vi "Puma_Ground_Control_Station_V2.0.vi"(0 "?":refnum<visa-resource-name>="COM4", 1 "?":u32=9600, 9 "XON":u8=17 format="%.0x", 14 "XOFF":u8=19 format="%.0x", 15 "?":u32=10000, 21 "?":bool=TRUE, 24 "?":u8=10 format="%.0x", 25 "bsize":u32=4096) -> ()   [LabVIEW 2015]
doc: "The Advanced Serial Read and Write example performs a Serial Port Read, a Serial Port Write, or a combination of these actions while setting some advanced serial features like buffer size, termination characters, and XON/XOFF flow control. The user selects the actions (read or write) on the front panel. If both are selected, the VI will write the data first, read the data and then close the VISA session that is opened to the port. \n\nThe parameters set for the serial port must match the parameters of the connected instrument or device. In this example, the bytes to read parameter specifies the number of bytes that the serial port reads. If there were more bytes at the port than the number specified in bytes to read, those bytes would not be read. Also, if you specify to read more bytes than the number of bytes actually read, you might receive a timeout error message.\n\nINSTRUCTIONS:\n1) Select the serial resource and configuration parameters (baud rate, data bits, parity, stop bits, flow control).\n2) Termination character can be enabled and set. Also, set the required input buffer size prior to running the example.\n3) Select the operations to be performed. \n4) Connect the serial port to your device. If no device is available, perform a loopback test by doing one of the following. Short pins 2 and 3 on a RS-232 cable or short pin 4 to pin 8 and pin 5 to pin 9 on a RS-485/422 cable. \n5) Run the VI to see the data read. (The \"read string\" will match the \"string to write\" if a loopback test was performed.)\n\nThis example exposes several advanced features that you may need for your application. Not all applications need all the features shown in this example. The input buffer size is likely an important setting that you want to control in your application. This example expands upon the flow control option for XON and XOFF, allowing the user to choose those control characters. The timeout parameter has been brought to the front panel so a user can specify the time period the VISA Read will wait for the number of bytes to read before timing out. Also, the user has several controls for the termination character, which is discussed later.\n\nNote that you can press the write and read buttons and change the bytes to read parameters on the fly, while the example is running. However, you must stop the example to change the other configuration parameters after the example has started running, and then run again.\n\nSet the I/O buffer size slightly higher the amount of data you expect to receive. This is very important for applications that don't use flow control, as you may lose characters if the receive buffer overflows.\n\nSetting the timeout period ensures that the operation returns with a timeout error if the operation cannot be performed in the specified time period. \n\nSome devices require a termination character in order to identify the end of command strings. Some devices send a termination character to signify the end of data to be read. \n\nThis example shows how you can end the Read operation once a termination character is detected in the buffer and/or append a termination character at the end of the Write data. To enable the Read to end on a termination character, use the VISA Configure Serial Port or use the VISA Properties Serial End Mode for Reads, Termination Character Enable, and Termination Character. To end the Write with a termination character, use the VISA Properties Serial End Mode for Writes, the Send End Enable, and Termination Character. In this example, the same termination character is used for both the Read and the Write. You can specify two different characters for your application, if desired.\n\nYour application may require specific characters for the XON/XOFF Flow Control. You can specify these characters with the VISA Properties Flow Control XOFF Character and Flow Control XON Character. Note that if the standard XON and XOFF characters are used, then decimal 17 and 19 are unavailable for data values. Remember that using flow control and setting an adequate buffer size allow you to prevent buffer overflows."
uses:
  <vilib>/Instr/_visa.llb/VISA Configure Serial Port (Instr).vi
panel:
  out "Reset Triggered":bool
  in  "PixHawk":bool
  in  "XON 2":u8=17 format="%.0x"
  in  "XOFF 2":u8=19 format="%.0x"
  in  "?":bool=TRUE
  in  "bsize 2":u32=4096
  in  "?":u8=10 format="%.0x"
  in  "?":bool=TRUE
  in  "?":u32=10000
  in  "?":refnum<visa-resource-name>="COM4"
  in  "?":u32=9600
  out "Max Values":T1={20.764332288, 0.0, 0.0, 0.0, 0.0, 0.0, 0.0, 201.058, 25.138999999999953, 0.0, 57.16000000000008, 0.0, 8.920000000000016, 15.403999999999996}
  in  "Data Filename":string
  out "Offset 7":dbl=-251.3
  out "Multiplier 7":dbl=1.264
  out "Offset 6":dbl=-250.2
  out "Offset 5":dbl=-250.3
  out "Offset 4":dbl=-1253.0
  out "Offset 3":dbl=-250.9
  out "Offset 2":dbl=-249.8
  out "Offset 1":dbl=-251.0
  out "Multiplier 6":dbl=1.264
  out "Multiplier 5":dbl=1.277
  out "Multiplier 4":dbl=6.36
  out "Multiplier 3":dbl=1.274
  out "Multiplier 2":dbl=1.267
  out "Multiplier 1":dbl=1.277
  out "Ready to Test":bool
  out "AV5-T Open":bool
  in  "Begin Checklist":bool
  out "Manual Abort Tested":bool
  out "Flight Control On":bool
  out "Reset Triggered 2":bool
  out "Primary Safety Active":bool
  out "Craft Triggered Softkill Active":bool
  out "Hardkill Active":bool
  out "ms":dbl=163640.0
  out "vcc 6":bool
  out "gnd 6":bool=TRUE
  out "TC6":bool
  out "vcc 5":bool
  out "gnd 5":bool=TRUE
  out "TC5":bool
  out "vcc 4":bool
  out "gnd 4":bool=TRUE
  out "TC4":bool
  out "vcc 3":bool
  out "gnd 3":bool=TRUE
  out "TC3":bool
  out "vcc 2":bool
  out "gnd 2":bool=TRUE
  out "TC2":bool
  out "vcc":bool
  out "gnd":bool=TRUE
  out "TC1":bool
  out "Motor 4":dbl=1000.0
  out "Motor 3":dbl=1000.0
  out "Motor 2":dbl=1000.0
  out "Motor 1":dbl=1000.0
  out "soft kill ind":bool
  out "dump fuel ind":bool
  out "abort ind":bool
  out "run ind":bool
  out "av6-t ind":bool
  out "Control input":bool
  out "return":bool
  out "Control (on/off)":bool
  out "PT5-M":dbl=-6.084000000000003
  out "PT2-M":dbl=-10.039999999999992
  out "PT2-U":dbl=-250.3
  out "PT1-U":dbl=-38.24000000000001
  out "PT3-M":dbl=-141.336
  out "PT1-M":dbl=9.934999999999945
  out "PT4-M":dbl=181.90299999999996
  out "TC6":dbl=-2.0
  out "TC5":dbl=-2.0
  out "TC4":dbl=-2.0
  out "TC3":dbl=-2.0
  out "TC2":dbl=-2.0
  out "TC1":dbl=-2.0
  out "Output":string="h:;"
  in  "?":enum32{"Ignore", "Test"}(tab)=enum."Test"
  in  "DValve / AV6-T":bool
  in  "Flight Control Board":bool
  in  "Safety":bool
  in  "Test Run":bool
  in  "Reset Control":bool
  in  "Primary Safety":bool
  out "?":bool
  in  "Primary Safety":bool
  in  "Soft Kill":bool
  in  "Simulate":bool
  in  "Reset FC":bool
  in  "Full Power":bool
  in  "Safety":bool
  in  "Takeoff":bool
  in  "Calibrate":bool
  in  "abort":bool
  out "?":dbl(graph)=20.40794784
  in  "Send":bool=TRUE
  in  "Recieve":bool=TRUE
  in  "bytes to read 2":u32=1000
  out "?":u32=107
  out "?":string[](array[string])=["339", "205", "86", "191", "0", "190", "194", "-2.00", "-2.00", "-2.00", "-2.00", "-2.00", "-2.00", "555", "1000", "1000", "1000", "1000", "163640"]
  out "?":string[](array[string])=["p:339,205,86,191,0,190,194", "t:-2.00,-2.00,-2.00,-2.00,-2.00,-2.00", "v:555", "m:1000,1000,1000,1000", "h:", "s:163640", ""]
  out "?":T1(graph)={20.40794784, -2.0, -2.0, -2.0, -2.0, -2.0, -2.0, 181.90299999999996, 9.934999999999945, -141.336, -38.24000000000001, -250.3, -10.039999999999992, -6.084000000000003}
  out "Voltage Sensor":dbl=20.40794784
  in  "dump fuel":bool
  in  "?":enum32{"PT", "TC", "Motors", "Ignore"}(tab)
  in  "?":T2(tab)
  out "PT 4":dbl(graph)=-38.24000000000001
  out "PT 5":dbl(graph)=-250.3
  out "PT 2":dbl(graph)=9.934999999999945
  out "PT 6":dbl(graph)=-10.039999999999992
  out "PT 3":dbl(graph)=-141.336
  out "PT 1":dbl(graph)=181.90299999999996
  out "PT 7":dbl(graph)=-6.084000000000003
  in  "?":T3(tab)
  out "TC 1":dbl(graph)=-2.0
  out "TC 2":dbl(graph)=-2.0
  out "TC 3":dbl(graph)=-2.0
  out "TC 4":dbl(graph)=-2.0
  out "TC 5":dbl(graph)=-2.0
  out "TC 6":dbl(graph)=-2.0
  out "Motors":cluster{dbl, dbl, dbl, dbl}(graph)={1000.0, 1000.0, 1000.0, 1000.0}
  out "?":bool=TRUE
  out "String":string
  in  "String 3":string
  in  "?":bool=TRUE
  in  "tank iso":bool
  in  "Av-6Tt":bool
  in  "FCU":bool
  in  "FOU":bool
  out "AV4-T":bool
  out "AV3-T":bool
  out "AV2-T":bool
  out "AV1-T":bool
  out "AV6-T":bool
  out "AV5-T":bool
  out "FO-U":bool
  out "FC-U":bool
  out "?":dbl(slide) scale=0.2..200.0
  # "green=open - check thermocouple attachments\nred=short gnd - contact Power or GNC\nblue=short vcc - contact Power or GNC"
  # "String Parsing Indicator"
  # "Data From Craft:"
  # "FC-U"
  # "FO-U"
  # "AV1-M"
  # "AV2-M"
  # "AV3-M"
  # "AV4-M"
  # "AV5-T"
  # "AV6-T"
  # "receive"
  # "send"
  # "Voltage"
  # "TCp2-M"
  # "Tcw1-E"
  # "TCp1-M"
  # "TCw4-E"
  # "TCw3-E"
  # "TCw2-E"
  # "PT4-M"
  # "PT1-M"
  # "PT3-M"
  # "PT1-U"
  # "PT2-U"
  # "PT2-M"
  # "PT5-M"
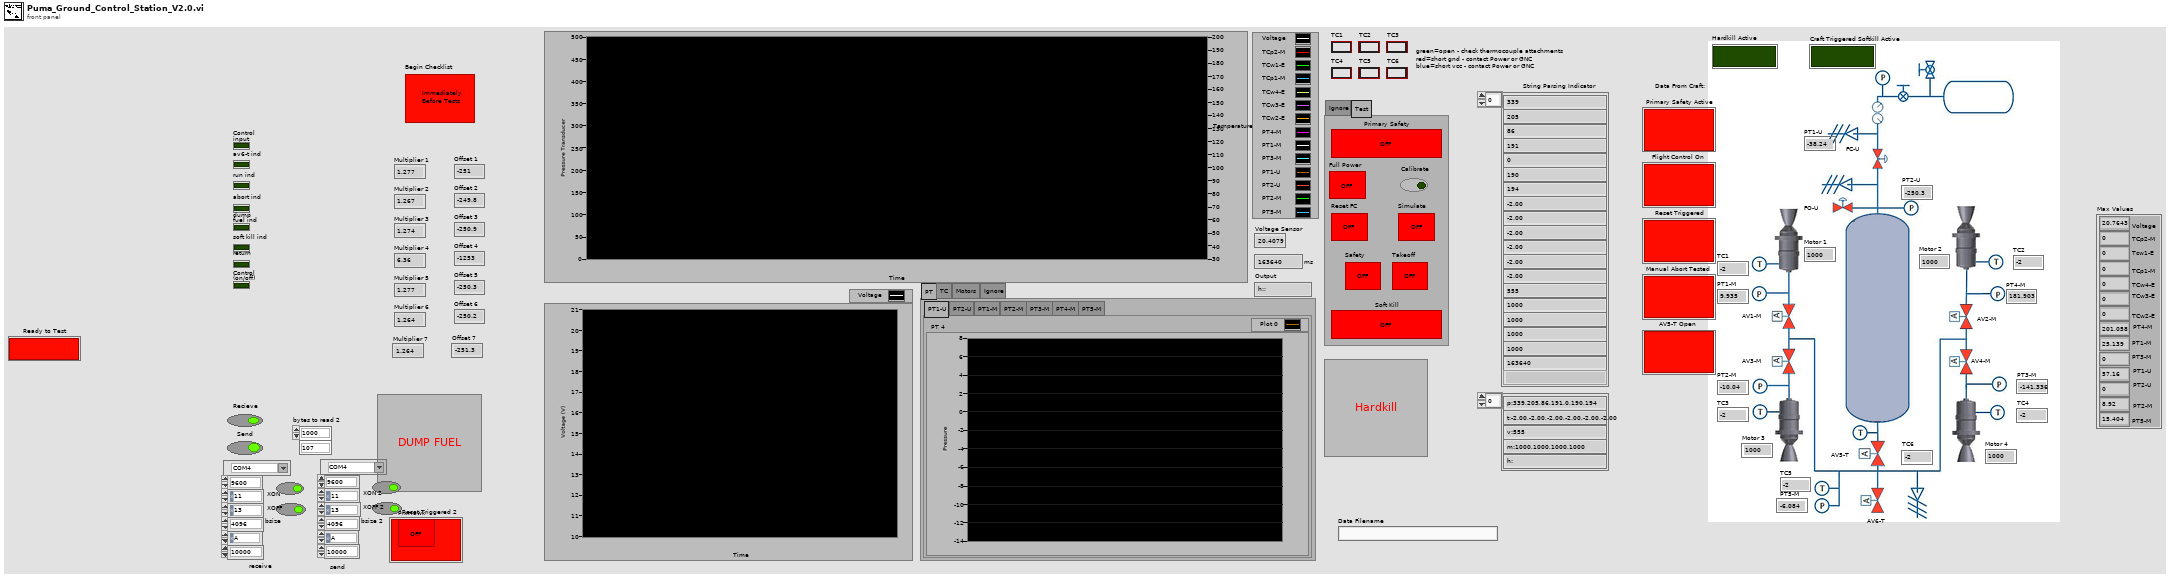
[diagram p1: front panel]
types:
  T1 = cluster{dbl, dbl, dbl, dbl, dbl, dbl, dbl, dbl, dbl, dbl, dbl, dbl, dbl, dbl}
  T2 = enum32{"PT1-U", "PT2-U", "PT1-M", "PT2-M", "PT3-M", "PT4-M", "PT5-M"}
  T3 = enum32{"TCp2-M", "TCw1-E", "TCp1-M", "TCw4-E", "TCw3-E", "TCw2-E"}
  T4 = enum16{"open", "replace", "create", "open or create", "replace or create", "replace or create with confirmation"}
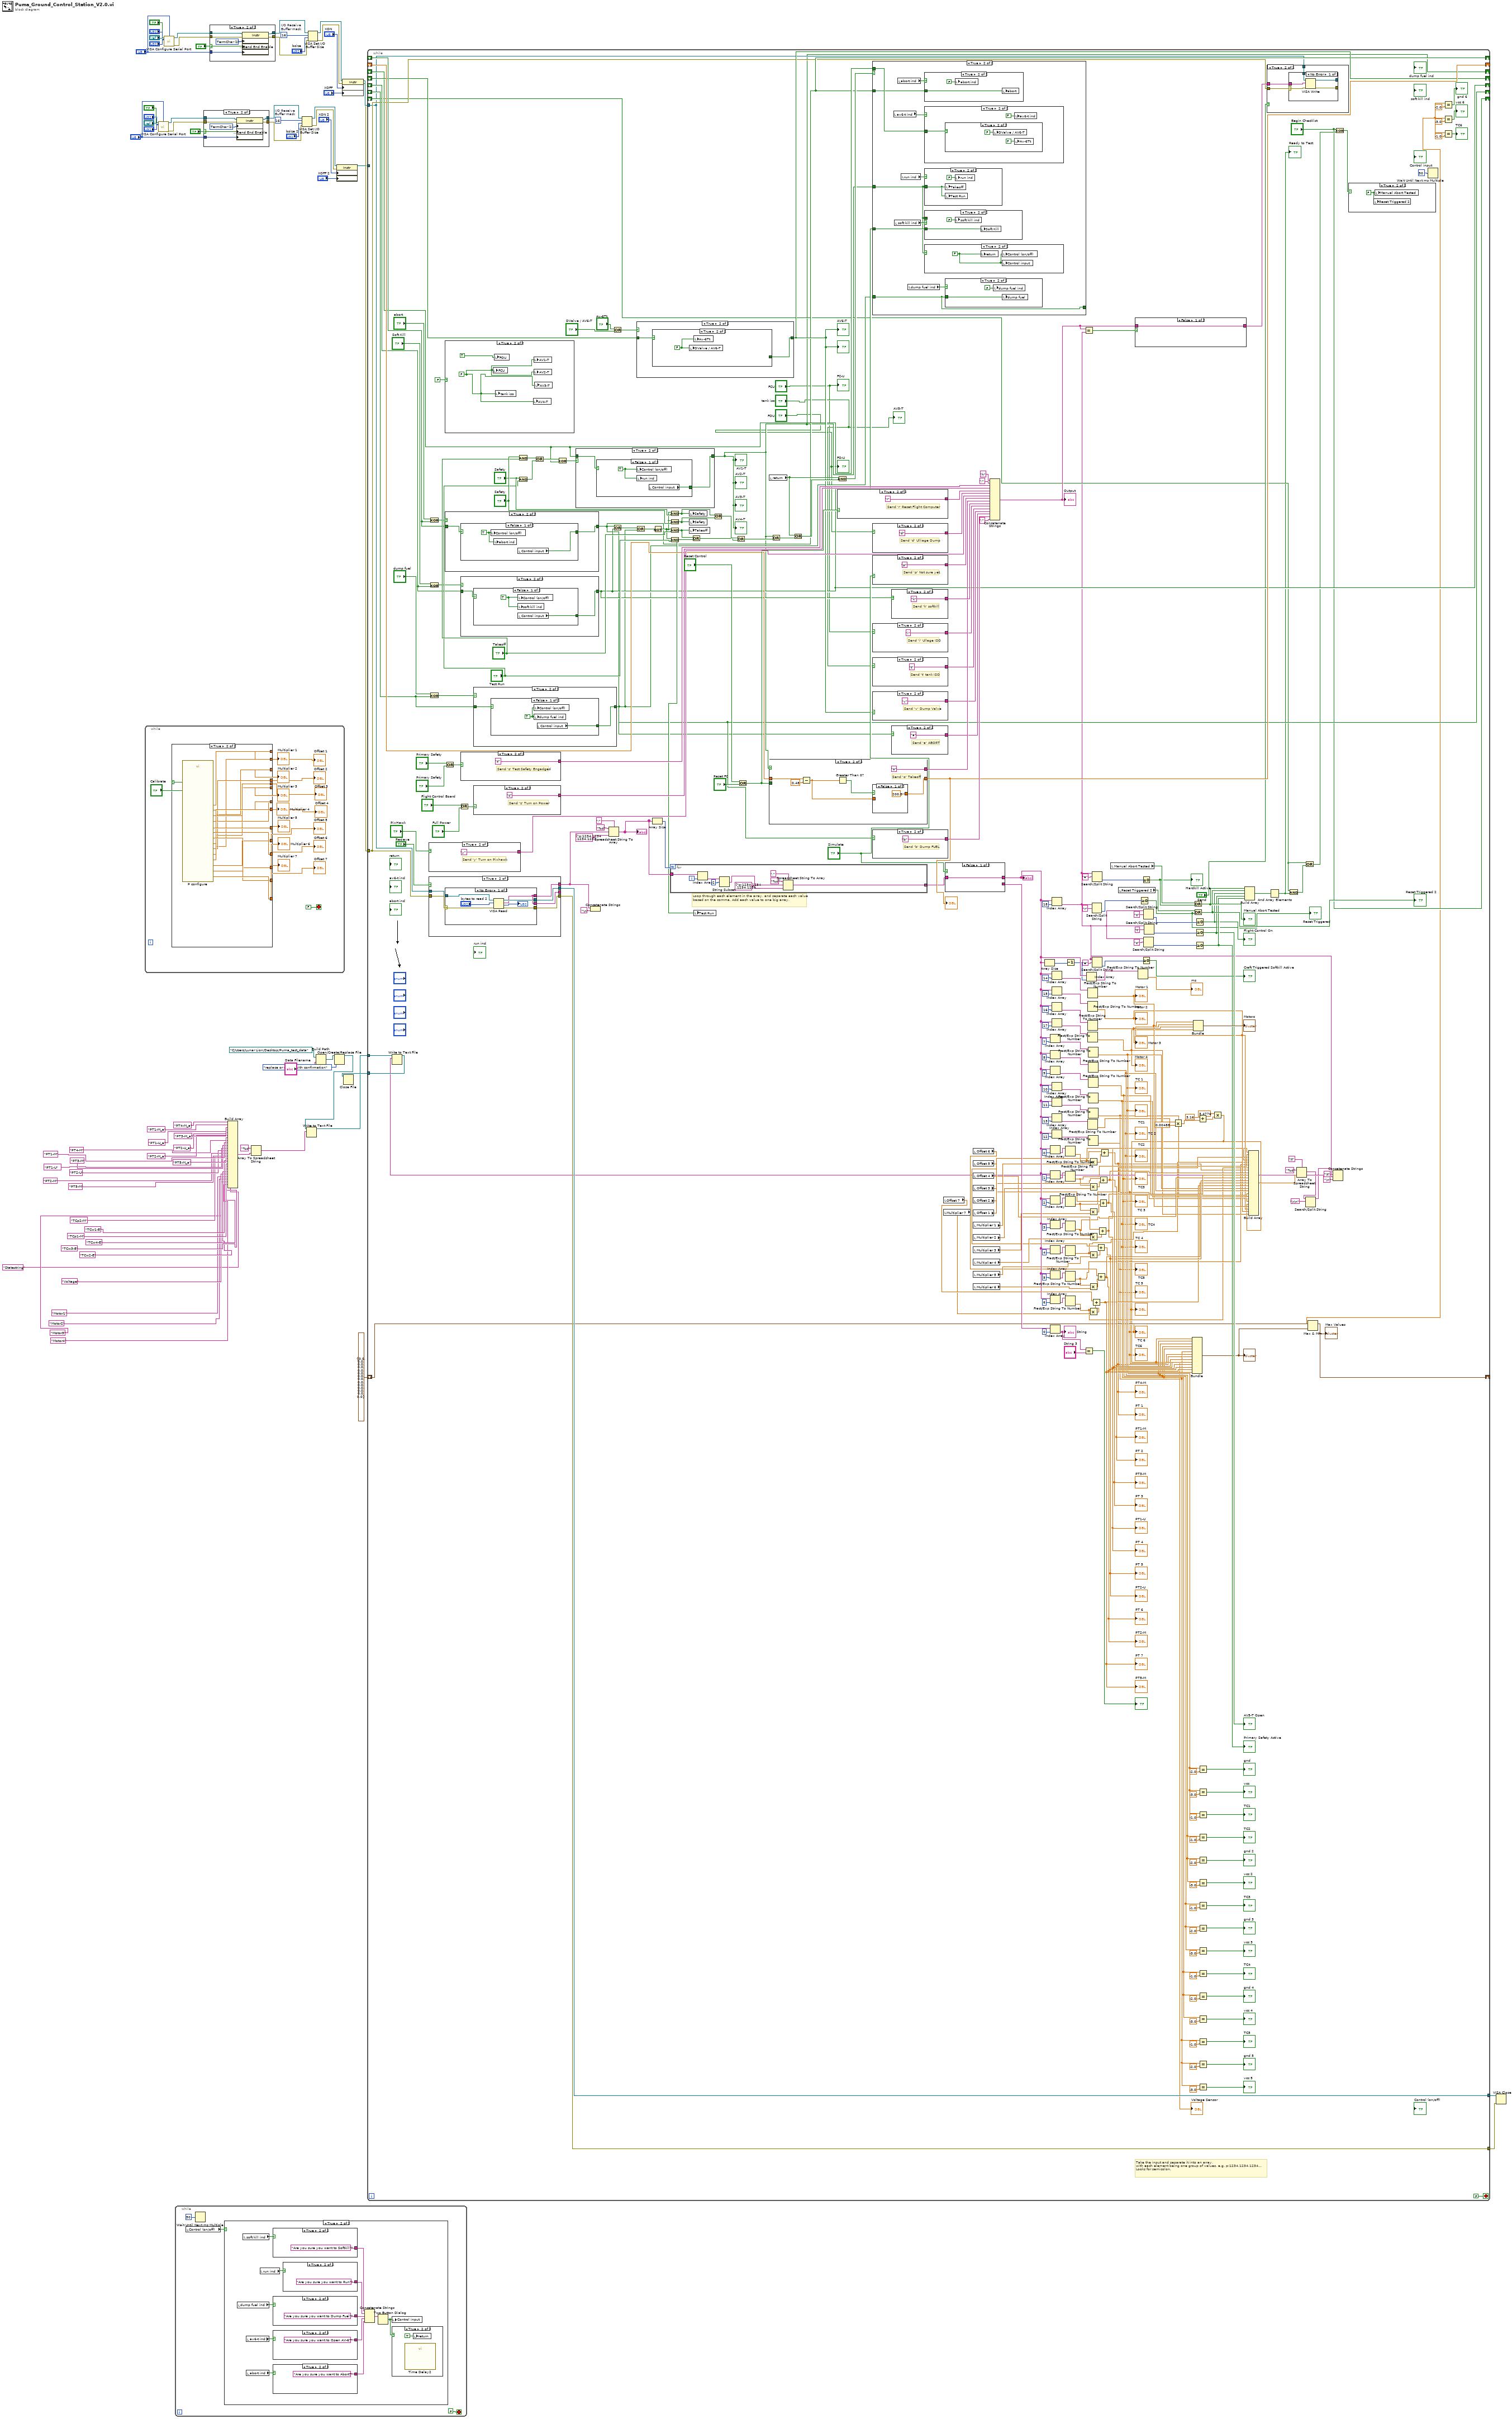
[diagram p0: block diagram]
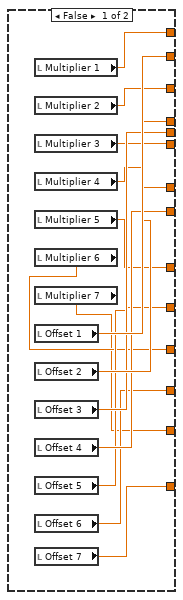
[diagram p3: hidden frame]
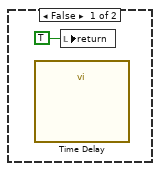
[diagram p10: hidden frame]
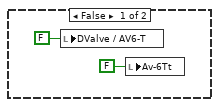
[diagram p16: hidden frame]
diagram:
  w44 = u16 16  # I/O Receive Buffer mask
  w70 = u16 16  # I/O Receive Buffer mask
  n1 = while {
    stop <- FALSE stop-if-true
    n2 = case shown="True" "Calibrate" {
      tunnel: [w104 w105] -> w88
      tunnel: [w103 w106] -> w87
      tunnel: [w102 w107] -> w86
      tunnel: [w101 w108] -> w85
      tunnel: [w99 w109] -> w80
      tunnel: [w100 w110] -> w84
      tunnel: [w98 w111] -> w83
      tunnel: [w97 w112] -> w75
      tunnel: [w96 w113] -> w79
      tunnel: [w95 w114] -> w76
      tunnel: [w94 w115] -> w77
      tunnel: [w93 w116] -> w82
      tunnel: [w92 w117] -> w81
      tunnel: [w91 w118] -> w78
      frame False {
        n3 = local read "Multiplier 1"() -> (w104:dbl)
        n4 = local read "Multiplier 2"() -> (w102:dbl)
        n5 = local read "Multiplier 3"() -> (w99:dbl)
        n6 = local read "Multiplier 4"() -> (w98:dbl)
        n7 = local read "Multiplier 5"() -> (w96:dbl)
        n8 = local read "Multiplier 6"() -> (w94:dbl)
        n9 = local read "Multiplier 7"() -> (w92:dbl)
        n10 = local read "Offset 1"() -> (w103:dbl)
        n11 = local read "Offset 2"() -> (w101:dbl)
        n12 = local read "Offset 3"() -> (w100:dbl)
        n13 = local read "Offset 4"() -> (w97:dbl)
        n14 = local read "Offset 5"() -> (w95:dbl)
        n15 = local read "Offset 6"() -> (w93:dbl)
        n16 = local read "Offset 7"() -> (w91:dbl)
      }
      frame True {
        n17 = call "P configure.vi"() -> ("Multiplier 1"=w105:dbl, "Offset 1"=w106:dbl, "Multiplier 2"=w107:dbl, "Offset 2"=w108:dbl, "Multiplier 3"=w109:dbl, "Offset 6"=w116:dbl, "Offset 3"=w110:dbl, "Offset 7"=w118:dbl, "Multiplier 4"=w111:dbl, "Multiplier 7"=w117:dbl, "Multiplier 6"=w115:dbl, "Offset 5"=w114:dbl, "Multiplier 5"=w113:dbl, "Offset 4"=w112:dbl)  [unwired: 2 in]
      }
    }
    "Multiplier 1" <- w88
    "Multiplier 2" <- w86
    "Multiplier 3" <- w80
    "Multiplier 4" <- w83
    "Multiplier 5" <- w79
    "Multiplier 6" <- w77
    "Offset 1" <- w87
    "Offset 2" <- w85
    "Offset 3" <- w84
    "Offset 4" <- w75
    "Offset 5" <- w76
    "Offset 6" <- w82
    "Multiplier 7" <- w81
    "Offset 7" <- w78
  }
  n18 = call-poly "VISA Configure Serial Port"("VISA resource name"="?", "timeout (10sec)"="?", "termination char\n(0xA = '\\n' = LF)"="?", "Enable Termination\nChar (T)"="?", "baud rate (9600)"="?") -> ("VISA resource name out"=w33:refnum<visa-resource-name>, "error out"=w36:errorcluster)  [unwired: 5 in, 4 out]
  n19 = call-poly "VISA Configure Serial Port"("VISA resource name"="?", "timeout (10sec)"="?", "termination char\n(0xA = '\\n' = LF)"="?", "Enable Termination\nChar (T)"="?", "baud rate (9600)"="?") -> ("VISA resource name out"=w59:refnum<visa-resource-name>, "error out"=w62:errorcluster)  [unwired: 5 in, 4 out]
  n20 = while {
    stop <- FALSE stop-if-true
    n21 = local read "Control (on/off)"() -> (w121:bool)
    n22 = Wait Until Next ms Multiple(millisecond multiple=u32 50 ("milliseconds to wait")) -> ()  [unwired: 1 out]
    n23 = case shown="True" w121 {
      frame False {
      }
      frame True {
        n24 = local read "dump fuel ind"() -> (w130:bool)
        n25 = local read "soft kill ind"() -> (w128:bool)
        n26 = local read "av6-t ind"() -> (w131:bool)
        n27 = local read "abort ind"() -> (w132:bool)
        n28 = local read "run ind"() -> (w129:bool)
        n29 = case shown="True" w128 {
          tunnel: [_ "Are you sure you want to Softkill?"] -> w123
          frame False {
          }
          frame True {
          }
        }
        n30 = case shown="True" w130 {
          tunnel: [_ "Are you sure you want to Dump Fuel?"] -> w125
          frame False {
          }
          frame True {
          }
        }
        n31 = case shown="True" w131 {
          tunnel: [_ "Are you sure you want to Open AV-6?"] -> w126
          frame False {
          }
          frame True {
          }
        }
        n32 = case shown="True" w132 {
          tunnel: [_ "Are you sure you want to Abort?"] -> w127
          frame False {
          }
          frame True {
          }
        }
        n33 = case shown="True" w129 {
          tunnel: [_ "Are you sure you want to Run?"] -> w124
          frame False {
          }
          frame True {
          }
        }
        n34 = Concatenate Strings(w123, w124, w125, w126, w127) -> (w122:string)
        n35 = Two Button Dialog(message=w122) -> (T button?=w133:bool)  [unwired: 2 in]
        n36 = local write "Control input"(w133) -> ()
        n37 = case shown="True" w133 {
          frame False {
            n38 = call "Time Delay"() -> ()  [unwired: 11 in, 1 out]
            n39 = local write "return"(TRUE) -> ()
          }
          frame True {
            n40 = call "Time Delay2"() -> ()  [unwired: 11 in, 1 out]
            n41 = local write "return"(TRUE) -> ()
          }
        }
      }
    }
  }
  n42 = case shown="True" "?" {
    selector: "?" -> [_ w143]
    tunnel: w33 -> [w141 w149]
    tunnel: w36 -> [w142 w148]
    tunnel: [w141 w147] -> w34
    tunnel: [w142 w146] -> w35
    tunnel: "?" -> [_ w144]
    frame False {
    }
    frame True {
      w145 = u16 2 items=["None", "LastBit", "TermChar", "Break"] ("Serial Settings:Serial End Mode for Writes")
      n43 = property class="Instr"(reference=w149, error in=w148, "Serial Settings:End Mode for Writes"=w145, "Message Based Settings:Send End Enable"=w143, "Message Based Settings:Termination Character"=w144) -> (reference out=w147:refnum<visa-resource-name>, error out=w146:errorcluster)
    }
  }
  n44 = case shown="True" "?" {
    selector: "?" -> [_ w152]
    tunnel: w59 -> [w150 w158]
    tunnel: w62 -> [w151 w157]
    tunnel: [w150 w156] -> w60
    tunnel: [w151 w155] -> w61
    tunnel: "?" -> [_ w153]
    frame False {
    }
    frame True {
      w154 = u16 2 items=["None", "LastBit", "TermChar", "Break"] ("Serial Settings:Serial End Mode for Writes")
      n45 = property class="Instr"(reference=w158, error in=w157, "Serial Settings:End Mode for Writes"=w154, "Message Based Settings:Send End Enable"=w152, "Message Based Settings:Termination Character"=w153) -> (reference out=w156:refnum<visa-resource-name>, error out=w155:errorcluster)
    }
  }
  n46 = Build Array("PT4-M_a", "PT1-M_a", "PT3-M_a", "PT1-U_a", "PT2-U_a", "PT2-M_a", "PT5-M_a", "PT4-M", "PT1-M", "PT3-M", "PT1-U", "PT2-U", "PT2-M", "PT5-M", "TCp2-M", "TCw1-E", "TCp1-M", "TCw4-E", "TCw3-E", "TCw2-E", "Voltage", "Motor1", "Motor2", "Motor3", "Motor4", "Statestring") -> (w5:string[])
  n47 = Array To Spreadsheet String(array=w5, 3:"%s" ("format string")) -> (spreadsheet string=w3:string)  [unwired: 1 in]
  n48 = VISA Set I/O Buffer Size(VISA resource name=w34, mask (16)=w44, size (4096)="bsize 2", error in (no error)=w35) -> (VISA resource name out=w40:refnum<visa-resource-name>, error out=w39:errorcluster)
  n49 = VISA Set I/O Buffer Size(VISA resource name=w60, mask (16)=w70, size (4096)="bsize", error in (no error)=w61) -> (VISA resource name out=w66:refnum<visa-resource-name>, error out=w65:errorcluster)
  n50 = Build Path(base path=path "C:/Users/Lunar Lion/Desktop/Puma_test_data" ("file path (use dialog)"), name or relative path="Data Filename") -> (appended path=w52:path)
  n51 = Open/Create/Replace File(file path (use dialog)=w52, operation (0:open)=T4."replace or create with confirmation") -> (refnum out=w2:refnum<file>)  [unwired: 4 in, 2 out]
  n52 = Write to Text File(file (use dialog)=w2, text=w3) -> (refnum out=w1:refnum<file>)  [unwired: 2 in, 2 out]
  n53 = property class="Instr"(reference=w40, error in=w39, "Serial Settings:Flow Control XON Character"="XON 2", "Serial Settings:Flow Control XOFF Character"="XOFF 2") -> (reference out=w32:refnum<visa-resource-name>)  [unwired: 1 out]
  n54 = property class="Instr"(reference=w66, error in=w65, "Serial Settings:Flow Control XON Character"="XON", "Serial Settings:Flow Control XOFF Character"="XOFF") -> (reference out=w58:refnum<visa-resource-name>, error out=w57:errorcluster)
  n55 = while {
    tunnel: w58 -> [w179]
    tunnel: w57 -> [w260]
    tunnel: [w400] -> w56
    tunnel: [w322] -> w55
    shift-right: [w372] -> _
    shift-left: _ -> [w371]
    shift-right: [w178] -> _
    shift-left: _ -> [w326]
    shift-right: [w334] -> _
    shift-left: _ -> [w335]
    shift-right: [w324] -> _
    shift-left: _ -> [w350]
    shift-right: [w325] -> _
    shift-left: _ -> [w347]
    shift-right: [w327] -> _
    shift-left: _ -> [w330]
    shift-right: ["Begin Checklist"] -> _
    shift-left: _ -> [w241]
    tunnel: w1 -> [w213]
    tunnel: [w210] -> w51
    shift-right: [w182] -> _
    shift-left: T1 {0.0, 0.0, 0.0, 0.0, 0.0, 0.0, 0.0, 0.0, 0.0, 0.0, 0.0, 0.0, 0.0, 0.0} -> [w181]
    tunnel: w32 -> [_]
    stop <- FALSE stop-if-true
    # "Loop through each element in the array, and separate each value\nbased on the comma. Add each value to one big array."
    # "Take the input and separate it into an array,\nwith each element being one group of values, e.g. p:1234,1234,1234...\nLooks for semicolon."
    n56 = case shown="True" "PixHawk" {
      tunnel: [_ "y" ("write buffer")] -> w393
      frame False {
      }
      frame True {
        # "Send 'y' Turn on Pixhawk"
      }
    }
    n57 = case shown="True" "Recieve" {
      tunnel: w260 -> [w526 w531]
      tunnel: w179 -> [w527 w530]
      tunnel: [w526 w533] -> w322
      tunnel: [w527 w532] -> w400
      tunnel: [_ w529] -> _
      tunnel: [_ w528] -> w212
      frame False {
      }
      frame True {
        n58 = case "Read bytes from port." shown="No Error" w531 {
          selector: w531 -> [w536 w541]
          tunnel: [w539 w541] -> w533
          tunnel: [w540 w542] -> w532
          tunnel: w530 -> [w537 w542]
          tunnel: [w534 _] -> w529
          tunnel: [w534 _] -> w528
          frame No Error {
            n59 = VISA Read(VISA resource name=w537, byte count="bytes to read 2", error in (no error)=w536) -> (VISA resource name out=w540:refnum<visa-resource-name>, read buffer=w534:string, return count=→"?":u32, error out=w539:errorcluster)
          }
          frame Error {
            # "Error occurred \nreading Bytes at \nSerial Port"
          }
        }
      }
    }
    n60 = Exclusive Or(1:w350, 2:"abort") -> (0:w352:bool)
    n61 = Exclusive Or(1:w330, 2:"Soft Kill") -> (0:w328:bool)
    n62 = Exclusive Or(1:w347, 2:"dump fuel") -> (0:w349:bool)
    n63 = Or(x="Primary Safety", y="Primary Safety") -> (x .or. y?=w368:bool)
    n64 = case shown="True" FALSE {
      frame False {
      }
      frame True {
        w432 = FALSE
        n65 = local write "FCU"(w432) -> ()
        n66 = local write "FOU"(TRUE) -> ()
        n67 = local write "tank iso"(w432) -> ()
        n68 = local write "AV4-T"(w432) -> ()
        n69 = local write "AV1-T"(w432) -> ()
        n70 = local write "AV2-T"(w432) -> ()
        n71 = local write "AV3-T"(w432) -> ()
      }
    }
    n72 = case shown="True" w352 {
      tunnel: [w478 w480] -> w324
      tunnel: w350 -> [w478 w479]
      frame False {
      }
      frame True {
        n73 = case shown="False" w479 {
          tunnel: [w481 FALSE ("T button?")] -> w480
          frame False {
            w482 = TRUE
            n74 = local write "Control (on/off)"(w482) -> ()
            n75 = local write "abort ind"(w482) -> ()
            n76 = local read "Control input"() -> (w481:bool)
          }
          frame True {
          }
        }
      }
    }
    n77 = Or(x="Flight Control Board", y="Full Power") -> (x .or. y?=w383:bool)
    n78 = case shown="True" w328 {
      tunnel: [w468 w470] -> w327
      tunnel: w330 -> [w468 w469]
      frame False {
      }
      frame True {
        n79 = case shown="False" w469 {
          tunnel: [w471 _] -> w470
          frame False {
            w472 = TRUE
            n80 = local write "Control (on/off)"(w472) -> ()
            n81 = local write "soft kill ind"(w472) -> ()
            n82 = local read "Control input"() -> (w471:bool)
          }
          frame True {
          }
        }
      }
    }
    n83 = case shown="True" w368 {
      tunnel: [_ "s" ("write buffer")] -> w397
      frame False {
      }
      frame True {
        # "Send 's' Test Safety Engadged"
      }
    }
    n84 = case shown="True" w349 {
      tunnel: [w473 w475] -> w325
      tunnel: w347 -> [w473 w474]
      frame False {
      }
      frame True {
        n85 = case shown="False" w474 {
          tunnel: [w477 _] -> w475
          frame False {
            w476 = TRUE
            n86 = local write "Control (on/off)"(w476) -> ()
            n87 = local write "dump fuel ind"(w476) -> ()
            n88 = local read "Control input"() -> (w477:bool)
          }
          frame True {
          }
        }
      }
    }
    n89 = case shown="True" w383 {
      tunnel: [_ "z" ("write buffer")] -> w396
      frame False {
      }
      frame True {
        # "Send 'z' Turn on Power"
      }
    }
    n90 = And(x="Safety", y="Takeoff") -> (x .and. y?=w386:bool)
    n91 = And(x="Safety", y="Test Run") -> (x .and. y?=w387:bool)
    n92 = Or(x=w386, y=w387) -> (x .or. y?=w355:bool)
    n93 = Exclusive Or(1:w326, 2:w355) -> (0:w354:bool)
    n94 = case shown="True" w354 {
      tunnel: [w484 w486] -> w178
      tunnel: w326 -> [w484 w485]
      frame False {
      }
      frame True {
        n95 = case shown="False" w485 {
          tunnel: [w488 _] -> w486
          frame False {
            w487 = TRUE
            n96 = local write "Control (on/off)"(w487) -> ()
            n97 = local write "run ind"(w487) -> ()
            n98 = local read "Control input"() -> (w488:bool)
          }
          frame True {
            w489 = FALSE
            n99 = local write "Control (on/off)"(w489) -> ()
            n100 = local write "Test Run"(w489) -> ()
            n101 = local write "Takeoff"(w489) -> ()
          }
        }
      }
    }
    "AV1-T" <- w178
    "AV4-T" <- w178
    "AV2-T" <- w178
    "AV3-T" <- w178
    n102 = Concatenate Strings(w212, "\n" ("string")) -> ()  [unwired: 1 out]
    n103 = Spreadsheet String To Array(delimiter (Tab)=";", format string="%d", spreadsheet string=w212, array type (2D Dbl)=string[] ["p:1234.1234.1234.1234,1234,1234", "t:1234,1234,1234"] ("Array of Strings 3")) -> (array=w426:string[])
    "?" <- w426
    n104 = Or(x="Av-6Tt", y="DValve / AV6-T") -> (x .or. y?=w331:bool)
    n105 = Or(x=w324, y=w327) -> (x .or. y?=w353:bool)
    n106 = Or(x=w353, y=w325) -> (x .or. y?=w319:bool)
    n107 = case shown="True" w331 {
      tunnel: [w462 w463] -> w334
      tunnel: w335 -> [w462 w464]
      frame False {
      }
      frame True {
        n108 = case shown="True" w464 {
          tunnel: [w466 _] -> w463
          frame False {
            w465 = TRUE
            n109 = local write "Control (on/off)"(w465) -> ()
            n110 = local write "av6-t ind"(w465) -> ()
            n111 = local read "Control input"() -> (w466:bool)
          }
          frame True {
            w467 = FALSE
            n112 = local write "DValve / AV6-T"(w467) -> ()
            n113 = local write "Av-6Tt"(w467) -> ()
          }
        }
      }
    }
    "AV6-T" <- w334
    "?" <- w334
    n114 = Array Size(array=w426) -> (size(s)=w427:i32)
    n115 = Not(x=w319) -> (.not. x?=w357:bool)
    n116 = And(x=w357, y="Safety") -> (x .and. y?=w339:bool)
    n117 = And(x=w357, y="Safety") -> (x .and. y?=w338:bool)
    n118 = And(x=w357, y="Takeoff") -> (x .and. y?=w337:bool)
    n119 = And(x=w357, y="Test Run") -> (x .and. y?=w336:bool)
    n120 = for {
      N: w427 -> [_]
      tunnel: w426 -> [w551]
      tunnel: [w543] -> w366 mode=concatenating
      i -> [w550]
      n121 = Index Array(array=w551, index=w550) -> (element=w546:string)
      n122 = String Subset(string=w546, offset (0)=2) -> (substring=w544:string)  [unwired: 1 in]
      n123 = Spreadsheet String To Array(delimiter (Tab)=",", format string="%d", spreadsheet string=w544, array type (2D Dbl)=string[] ["p:1234.1234.1234.1234,1234,1234", "t:1234,1234,1234"] ("Array of Strings 3")) -> (array=w543:string[])
    }
    n124 = local write "Safety"(w339) -> ()
    n125 = local write "Safety"(w338) -> ()
    n126 = local write "Takeoff"(w337) -> ()
    n127 = Or(x=w337, y=w336) -> (x .or. y?=w341:bool)
    n128 = local write "Test Run"(w336) -> ()
    n129 = Or(x=w339, y=w338) -> (x .or. y?=w342:bool)
    n130 = Or(x=w342, y=w341) -> (x .or. y?=w340:bool)
    n131 = Or(x="Reset Control", y="Reset FC") -> (x .or. y?=w373:bool)
    n132 = local read "return"() -> (w345:bool)
    n133 = case shown="True" w178 {
      tunnel: [_ "o" ("write buffer")] -> w391
      tunnel: w371 -> [w501 w509]
      tunnel: [w502 w505] -> w372
      tunnel: w373 -> [w500 _]
      frame False {
        n134 = case shown="False" w500 {
          tunnel: [w503 200.0] -> w502
          tunnel: w501 -> [w503 _]
          frame False {
          }
          frame True {
          }
        }
      }
      frame True {
        # "Send 'o' Takeoff"
        n135 = Subtract(x=w509, y=0.48) -> (x-y=w506:dbl)
        n136 = Greater Than 0?(x=w506) -> (x > 0?=w507:bool)
        n137 = case shown="False" w507 {
          tunnel: w506 -> [_ w512]
          tunnel: [200.0 w512] -> w505
          frame False {
          }
          frame True {
          }
        }
      }
    }
    "?" <- w372
    n138 = Or(x=w178, y=w340) -> (x .or. y?=w343:bool)
    n139 = Or(x=w345, y=w343) -> (x .or. y?=w346:bool)
    n140 = case shown="True" w373 {
      tunnel: [_ "r" ("write buffer")] -> w395
      frame False {
      }
      frame True {
        # "Send 'r' Reset Flight Computer"
      }
    }
    n141 = And(x=w345, y=w346) -> (x .and. y?=w344:bool)
    n142 = case shown="True" w344 {
      tunnel: w178 -> [_ w437]
      tunnel: w327 -> [_ w440]
      tunnel: w326 -> [_ w439]
      tunnel: [_ w438] -> _
      tunnel: w325 -> [_ w438]
      tunnel: w324 -> [_ w436]
      frame False {
      }
      frame True {
        n143 = local read "av6-t ind"() -> (w441:bool)
        n144 = local read "soft kill ind"() -> (w445:bool)
        n145 = local read "abort ind"() -> (w442:bool)
        n146 = local read "run ind"() -> (w443:bool)
        n147 = local read "dump fuel ind"() -> (w444:bool)
        n148 = case shown="True" w442 {
          tunnel: w436 -> [_ w452]
          frame False {
          }
          frame True {
            n149 = local write "abort ind"(FALSE) -> ()
            n150 = local write "abort"(w452) -> ()
          }
        }
        n151 = case shown="True" w441 {
          tunnel: w439 -> [_ w447]
          frame False {
          }
          frame True {
            n152 = case shown="True" w447 {
              frame False {
                n153 = local write "DValve / AV6-T"(FALSE) -> ()
                n154 = local write "Av-6Tt"(FALSE) -> ()
              }
              frame True {
                n155 = local write "DValve / AV6-T"(FALSE) -> ()
                n156 = local write "Av-6Tt"(FALSE) -> ()
              }
            }
            n157 = local write "av6-t ind"(FALSE) -> ()
          }
        }
        n158 = case shown="True" w443 {
          tunnel: w437 -> [_ w459]
          frame False {
          }
          frame True {
            n159 = local write "Takeoff"(w459) -> ()
            n160 = local write "Test Run"(w459) -> ()
            n161 = local write "run ind"(FALSE) -> ()
          }
        }
        n162 = case shown="True" w445 {
          tunnel: w437 -> [_ _]
          tunnel: w440 -> [_ w454]
          frame False {
          }
          frame True {
            n163 = local write "soft kill ind"(FALSE) -> ()
            n164 = local write "Soft Kill"(w454) -> ()
          }
        }
        n165 = case shown="True" w437 {
          frame False {
            w460 = FALSE
            n166 = local write "return"(w460) -> ()
            n167 = local write "Control (on/off)"(w460) -> ()
            n168 = local write "Control input"(w460) -> ()
          }
          frame True {
            w461 = FALSE
            n169 = local write "return"(w461) -> ()
            n170 = local write "Control (on/off)"(w461) -> ()
            n171 = local write "Control input"(w461) -> ()
          }
        }
        n172 = case shown="True" w444 {
          tunnel: w438 -> [_ w456]
          frame False {
          }
          frame True {
            n173 = local write "dump fuel ind"(FALSE) -> ()
            n174 = local write "dump fuel"(w456) -> ()
          }
        }
      }
    }
    n175 = case shown="True" "FOU" {
      tunnel: [_ "d" ("write buffer")] -> w382
      frame False {
      }
      frame True {
        # "Send 'd' Ulliage Dump"
      }
    }
    n176 = case shown="True" "Simulate" {
      tunnel: [_ "p" ("write buffer")] -> w392
      frame False {
      }
      frame True {
        # "Send 'p' Not sure yet"
      }
    }
    n177 = case shown="True" "FCU" {
      tunnel: [_ "i" ("write buffer")] -> w381
      frame False {
      }
      frame True {
        # "Send 'i' Ullage ISO"
      }
    }
    n178 = case shown="True" "tank iso" {
      tunnel: [_ "t" ("write buffer")] -> w380
      frame False {
      }
      frame True {
        # "Send 't' tank ISO"
      }
    }
    n179 = case shown="True" w334 {
      tunnel: [_ "v" ("write buffer")] -> w379
      frame False {
      }
      frame True {
        # "Send 'v' Dump Valve"
      }
    }
    n180 = case shown="True" w325 {
      tunnel: [_ "b" ("write buffer")] -> w378
      frame False {
      }
      frame True {
        # "Send 'b' Dump FUEL"
      }
    }
    n181 = case shown="True" w327 {
      tunnel: [_ "k" ("write buffer")] -> w394
      frame False {
      }
      frame True {
        # "Send 'k' softkill"
      }
    }
    n182 = case shown="True" w324 {
      tunnel: [_ "a" ("write buffer")] -> w377
      frame False {
      }
      frame True {
        # "Send 'a' ABORT"
      }
    }
    n183 = local read "Offset 7"() -> (w216:dbl)
    n184 = local read "Multiplier 7"() -> (w215:dbl)
    n185 = case shown="False" "Simulate" {
      tunnel: w366 -> [w490 w491]
      tunnel: [w490 w491] -> w264
      tunnel: [_ w491] -> w365
      frame False {
      }
      frame True {
      }
    }
    "?" <- w264
    n186 = local read "Offset 6"() -> (w218:dbl)
    n187 = local read "Offset 5"() -> (w219:dbl)
    n188 = local read "Offset 4"() -> (w221:dbl)
    n189 = local read "Offset 3"() -> (w223:dbl)
    n190 = local read "Offset 2"() -> (w225:dbl)
    n191 = local read "Offset 1"() -> (w227:dbl)
    n192 = local read "Multiplier 1"() -> (w228:dbl)
    n193 = local read "Multiplier 2"() -> (w226:dbl)
    n194 = local read "Multiplier 3"() -> (w224:dbl)
    n195 = local read "Multiplier 4"() -> (w222:dbl)
    n196 = local read "Multiplier 5"() -> (w220:dbl)
    n197 = local read "Multiplier 6"() -> (w217:dbl)
    n198 = Concatenate Strings("h" ("string"), ":" ("string"), w397, w396, w395, w382, w393, w392, w391, w394, w381, w380, w379, w377, w378, ";" ("string")) -> (w314:string)
    "Output" <- w314
    n199 = Array Size(array=w264) -> (size(s)=w263:i32)
    n200 = Index Array(array=w264, index=7) -> (element=w408:string)
    n201 = Index Array(array=w264, index=8) -> (element=w407:string)
    n202 = Index Array(array=w264, index=9) -> (element=w406:string)
    n203 = Index Array(array=w264, index=0) -> (element=w419:string)
    n204 = Index Array(array=w264, index=1) -> (element=w418:string)
    n205 = Index Array(array=w264, index=2) -> (element=w417:string)
    n206 = Index Array(array=w264, index=3) -> (element=w416:string)
    n207 = Index Array(array=w264, index=4) -> (element=w415:string)
    n208 = Index Array(array=w264, index=5) -> (element=w414:string)
    n209 = Index Array(array=w264, index=6) -> (element=w375:string)
    n210 = Index Array(array=w365, index=0) -> (element=w364:string)
    "String" <- w364
    n211 = Index Array(array=w264, index=18) -> (element=w193:string)
    n212 = Index Array(array=w264, index=14) -> (element=w309:string)
    n213 = Index Array(array=w264, index=15) -> (element=w308:string)
    n214 = Index Array(array=w264, index=16) -> (element=w307:string)
    n215 = Index Array(array=w264, index=17) -> (element=w306:string)
    n216 = Index Array(array=w264, index=10) -> (element=w404:string)
    n217 = Index Array(array=w264, index=11) -> (element=w403:string)
    n218 = Index Array(array=w264, index=13) -> (element=w398:string)
    n219 = Index Array(array=w264, index=12) -> (element=w402:string)
    n220 = Fract/Exp String To Number(string=w419) -> (number=w189:dbl)  [unwired: 3 in, 1 out]
    n221 = Fract/Exp String To Number(string=w418) -> (number=w188:dbl)  [unwired: 3 in, 1 out]
    n222 = Fract/Exp String To Number(string=w417) -> (number=w187:dbl)  [unwired: 3 in, 1 out]
    n223 = Fract/Exp String To Number(string=w416) -> (number=w186:dbl)  [unwired: 3 in, 1 out]
    n224 = Fract/Exp String To Number(string=w415) -> (number=w185:dbl)  [unwired: 3 in, 1 out]
    n225 = Fract/Exp String To Number(string=w414) -> (number=w184:dbl)  [unwired: 3 in, 1 out]
    n226 = Fract/Exp String To Number(string=w375) -> (number=w183:dbl)  [unwired: 3 in, 1 out]
    n227 = Decrement(x=w263) -> (x-1=w262:i32)
    n228 = Equal?(x=w314, y=w193) -> (x = y?=w316:bool)
    n229 = Equal?(x=w364, y="String 3") -> (x = y?=→"?":bool)
    n230 = Index Array(array=w264, index=w262) -> (element=w267:string)
    n231 = Fract/Exp String To Number(string=w309) -> (number=w199:dbl)  [unwired: 3 in, 1 out]
    "Motor 1" <- w199
    n232 = Fract/Exp String To Number(string=w308) -> (number=w198:dbl)  [unwired: 3 in, 1 out]
    "Motor 2" <- w198
    n233 = Fract/Exp String To Number(string=w307) -> (number=w305:dbl)  [unwired: 3 in, 1 out]
    "Motor 3" <- w305
    n234 = Fract/Exp String To Number(string=w306) -> (number=w197:dbl)  [unwired: 3 in, 1 out]
    "Motor 4" <- w197
    n235 = Fract/Exp String To Number(string=w398) -> (number=w176:dbl)  [unwired: 3 in, 1 out]
    n236 = Fract/Exp String To Number(string=w408) -> (number=w203:dbl)  [unwired: 3 in, 1 out]
    "TC 1" <- w203
    "TC1" <- w203
    n237 = Fract/Exp String To Number(string=w407) -> (number=w202:dbl)  [unwired: 3 in, 1 out]
    "TC 2" <- w202
    "TC2" <- w202
    n238 = Fract/Exp String To Number(string=w406) -> (number=w201:dbl)  [unwired: 3 in, 1 out]
    "TC 3" <- w201
    "TC3" <- w201
    n239 = Fract/Exp String To Number(string=w404) -> (number=w200:dbl)  [unwired: 3 in, 1 out]
    "TC 4" <- w200
    "TC4" <- w200
    n240 = Fract/Exp String To Number(string=w403) -> (number=w168:dbl)  [unwired: 3 in, 1 out]
    "TC 5" <- w168
    "TC5" <- w168
    n241 = Fract/Exp String To Number(string=w402) -> (number=w169:dbl)  [unwired: 3 in, 1 out]
    "TC 6" <- w169
    "TC6" <- w169
    n242 = Multiply(x=w189, y=w228) -> (x*y=w235:dbl)
    n243 = Multiply(x=w188, y=w226) -> (x*y=w234:dbl)
    n244 = Multiply(x=w187, y=w224) -> (x*y=w233:dbl)
    n245 = Multiply(x=w186, y=w222) -> (x*y=w232:dbl)
    n246 = Multiply(x=w185, y=w220) -> (x*y=w231:dbl)
    n247 = Multiply(x=w184, y=w217) -> (x*y=w230:dbl)
    n248 = Multiply(x=w183, y=w215) -> (x*y=w229:dbl)
    n249 = Add(x=w216, y=w229) -> (x+y=w204:dbl)
    "PT5-M" <- w204
    "PT 7" <- w204
    n250 = Search/Split String(string=w193, search string/char (-)="r") -> (offset of match=w252:i32)  [unwired: 1 in, 2 out]
    n251 = Search/Split String(string=w193, search string/char (-)="a") -> (offset of match=w259:i32)  [unwired: 1 in, 2 out]
    n252 = Search/Split String(string=w193, search string/char (-)="e") -> (offset of match=w320:i32)  [unwired: 1 in, 2 out]
    n253 = Add(x=w219, y=w231) -> (x+y=w206:dbl)
    "PT 5" <- w206
    "PT2-U" <- w206
    n254 = Add(x=w218, y=w230) -> (x+y=w205:dbl)
    "PT 6" <- w205
    "PT2-M" <- w205
    n255 = Add(x=w221, y=w232) -> (x+y=w207:dbl)
    "PT 4" <- w207
    "PT1-U" <- w207
    n256 = Add(x=w223, y=w233) -> (x+y=w208:dbl)
    "PT 3" <- w208
    "PT3-M" <- w208
    n257 = Add(x=w225, y=w234) -> (x+y=w209:dbl)
    "PT 2" <- w209
    "PT1-M" <- w209
    n258 = Add(x=w227, y=w235) -> (x+y=w164:dbl)
    "PT 1" <- w164
    "PT4-M" <- w164
    n259 = local read "Manual Abort Tested"() -> (w249:bool)
    n260 = local read "Reset Triggered 2"() -> (w250:bool)
    n261 = case shown="False" w316 {
      tunnel: [w435 _] -> w315
      tunnel: w314 -> [w435 _]
      frame False {
      }
      frame True {
      }
    }
    n262 = Fract/Exp String To Number(string=w267) -> (number=→"ms":dbl)  [unwired: 3 in, 1 out]
    n263 = Greater Or Equal To 0?(x=w252) -> (x >= 0?=w177:bool)
    "Reset Triggered" <- w177
    n264 = Greater Or Equal To 0?(x=w259) -> (x >= 0?=w160:bool)
    "Hardkill Active" <- w160
    n265 = Greater Or Equal To 0?(x=w320) -> (x >= 0?=→"Craft Triggered Softkill Active":bool)
    n266 = Search/Split String(string=w193, search string/char (-)="z") -> (offset of match=w254:i32)  [unwired: 1 in, 2 out]
    n267 = Search/Split String(string=w193, search string/char (-)="s") -> (offset of match=w256:i32)  [unwired: 1 in, 2 out]
    n268 = Search/Split String(string=w193, search string/char (-)="t") -> (offset of match=w248:i32)  [unwired: 1 in, 2 out]
    n269 = Multiply(x=w176, y=0.00488) -> (x*y=w174:dbl)
    n270 = Or(x=w249, y=w160) -> (x .or. y?=w246:bool)
    "Manual Abort Tested" <- w246
    n271 = Or(x=w250, y=w177) -> (x .or. y?=w245:bool)
    "Reset Triggered 2" <- w245
    n272 = Bundle(w199, w198, w305, w197) -> (→"Motors":cluster{dbl, dbl, dbl, dbl})  [unwired: 1 in]
    n273 = Greater Or Equal To 0?(x=w254) -> (x >= 0?=w214:bool)
    "Flight Control On" <- w214
    n274 = Greater Or Equal To 0?(x=w248) -> (x >= 0?=w243:bool)
    "AV5-T Open" <- w243
    n275 = Greater Or Equal To 0?(x=w256) -> (x >= 0?=w244:bool)
    "Primary Safety Active" <- w244
    n276 = Add(x=3.16, y=w174) -> (x+y=w172:dbl)
    n277 = Equal?(x=w203, y=-2.0) -> (x = y?=→"gnd":bool)
    n278 = Equal?(x=w203, y=-3.0) -> (x = y?=→"vcc":bool)
    n279 = Equal?(x=w203, y=-1.0) -> (x = y?=→"TC1":bool)
    n280 = Equal?(x=w202, y=-1.0) -> (x = y?=→"TC2":bool)
    n281 = Equal?(x=w202, y=-2.0) -> (x = y?=→"gnd 2":bool)
    n282 = Equal?(x=w202, y=-3.0) -> (x = y?=→"vcc 2":bool)
    n283 = Equal?(x=w201, y=-1.0) -> (x = y?=→"TC3":bool)
    n284 = Equal?(x=w201, y=-2.0) -> (x = y?=→"gnd 3":bool)
    n285 = Equal?(x=w201, y=-3.0) -> (x = y?=→"vcc 3":bool)
    n286 = Equal?(x=w200, y=-1.0) -> (x = y?=→"TC4":bool)
    n287 = Equal?(x=w200, y=-2.0) -> (x = y?=→"gnd 4":bool)
    n288 = Equal?(x=w200, y=-3.0) -> (x = y?=→"vcc 4":bool)
    n289 = Equal?(x=w168, y=-1.0) -> (x = y?=→"TC5":bool)
    n290 = Equal?(x=w168, y=-2.0) -> (x = y?=→"gnd 5":bool)
    n291 = Equal?(x=w168, y=-3.0) -> (x = y?=→"vcc 5":bool)
    n292 = Multiply(x=3.4776, y=w172) -> (x*y=w170:dbl)
    "Voltage Sensor" <- w170
    "?" <- w170
    n293 = Bundle(w170, w203, w202, w201, w200, w168, w169, w164, w209, w208, w207, w206, w205, w204) -> (w180:T1)  [unwired: 1 out]
    "?" <- w180
    n294 = Build Array(w246, w245, w214, w243, w244) -> (w242:bool[])
    n295 = Build Array(w189, w188, w187, w186, w185, w184, w183, w164, w209, w208, w207, w206, w205, w204, w203, w202, w201, w200, w168, w169, w170, w199, w198, w198, w197) -> (w196:dbl[])
    n296 = case shown="True" "Send" {
      tunnel: w260 -> [_ w519]
      tunnel: w315 -> [_ w518]
      tunnel: w179 -> [_ w517]
      frame False {
      }
      frame True {
        n297 = case shown="No Error" w519 {
          selector: w519 -> [w522 w525]
          tunnel: [w524 _] -> _
          tunnel: [w523 w525] -> _
          tunnel: w518 -> [w521 _]
          tunnel: w517 -> [w520 _]
          frame No Error {
            n298 = VISA Write(VISA resource name=w520, write buffer=w521, error in (no error)=w522) -> (VISA resource name out=w524:refnum<visa-resource-name>, error out=w523:errorcluster)  [unwired: 1 out]
          }
          frame Error {
          }
        }
      }
    }
    n299 = And Array Elements(Boolean array=w242) -> (logical AND=w238:bool)
    "Ready to Test" <- w238
    n300 = And(x=w241, y=w238) -> (x .and. y?=w240:bool)
    n301 = Array To Spreadsheet String(delimiter (Tab)="\t", array=w196, 3:"%d" ("format string")) -> (spreadsheet string=w167:string)
    n302 = Or(x=w241, y=w240) -> (x .or. y?=w239:bool)
    n303 = Search/Split String(string=w167, search string/char (-)="\r\n") -> (substring before match=w165:string)  [unwired: 1 in, 2 out]
    n304 = Max & Min(x=w181, y=w180) -> (max(x,y)=w182:T1)  [unwired: 1 out]
    "Max Values" <- w182
    n305 = Concatenate Strings(w165, "\t" ("string"), w193, "\n" ("string")) -> (w191:string)
    n306 = Write to Text File(file (use dialog)=w213, text=w191) -> (refnum out=w210:refnum<file>)  [unwired: 2 in, 2 out]
    n307 = Exclusive Or(1:w239, 2:"Begin Checklist") -> (0:w257:bool)
    n308 = case shown="True" w257 {
      frame False {
      }
      frame True {
        w434 = FALSE
        n309 = local write "Reset Triggered 2"(w434) -> ()
        n310 = local write "Manual Abort Tested"(w434) -> ()
      }
    }
    n311 = Wait Until Next ms Multiple(millisecond multiple=u32 50 ("milliseconds to wait")) -> ()  [unwired: 1 out]
    n312 = Equal?(x=w169, y=-2.0) -> (x = y?=→"gnd 6":bool)
    n313 = Equal?(x=w169, y=-3.0) -> (x = y?=→"vcc 6":bool)
    n314 = Equal?(x=w169, y=-1.0) -> (x = y?=→"TC6":bool)
    "FO-U" <- "FOU"
    "AV5-T" <- "tank iso"
    "FC-U" <- "FCU"
  }
  n315 = Close File(refnum=w51) -> ()  [unwired: 1 in, 2 out]
  n316 = VISA Close(VISA resource name=w56, error in (no error)=w55) -> ()  [unwired: 1 out]
